vi "Z_MN_4952.vi"(4 "u":dbl format="%#_13g") -> (1 "y":dbl)   [LabVIEW 2019]
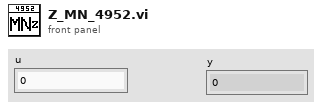
[diagram p1: front panel]
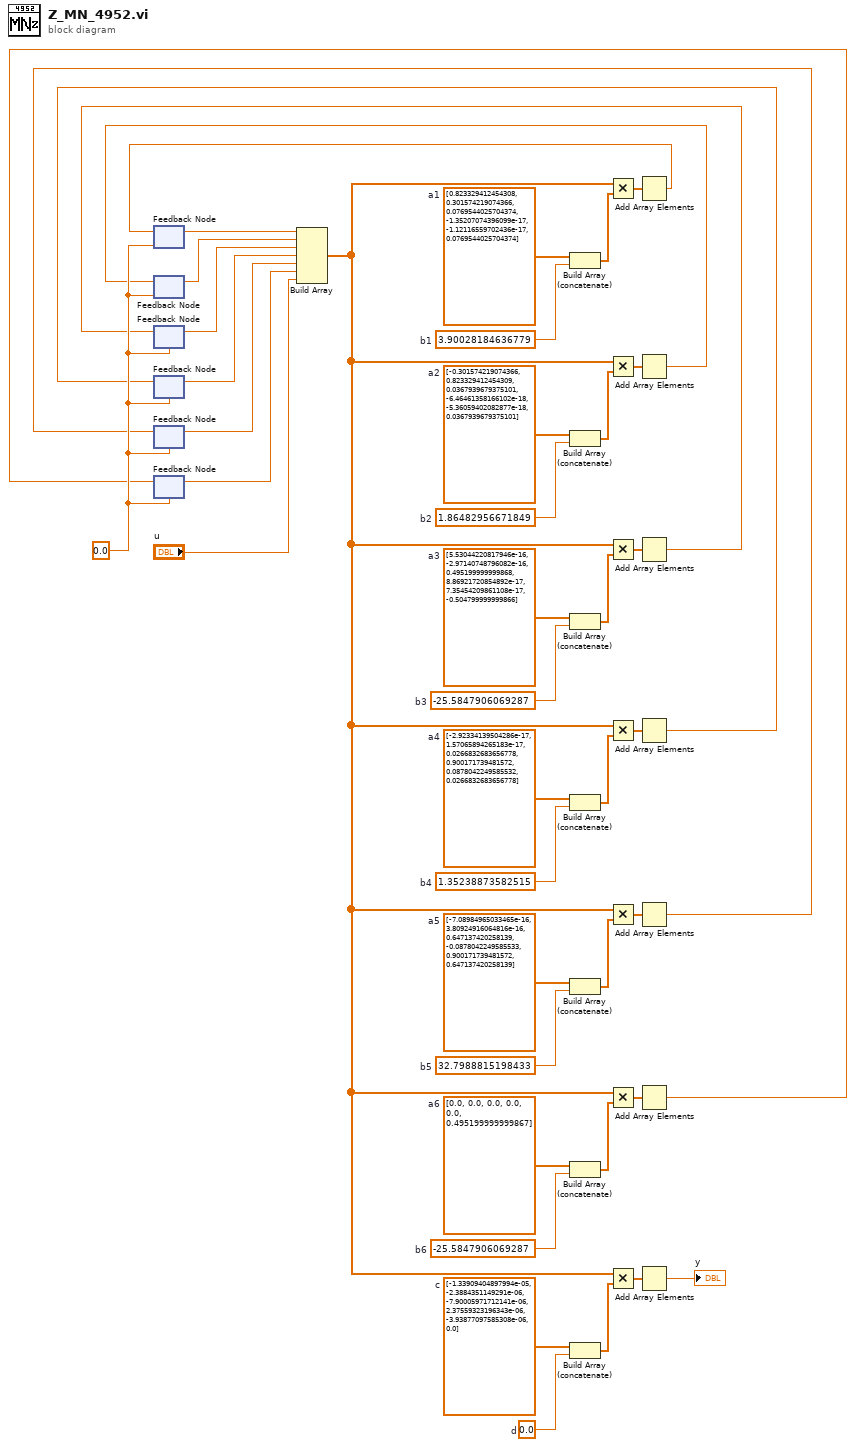
[diagram p0: block diagram]
diagram:
  w3 = 0.0  # d
  w2 = dbl[] [-1.33909404897994e-05, -2.3884351149291e-06, -7.90005971712141e-06, 2.37559323196343e-06, -3.93877097585308e-06, 0.0]  # c
  w5 = -25.5847906069287  # b6
  w6 = dbl[] [0.0, 0.0, 0.0, 0.0, 0.0, 0.495199999999867]  # a6
  w9 = 32.7988815198433  # b5
  w8 = dbl[] [-7.08984965033465e-16, 3.80924916064816e-16, 0.647137420258139, -0.0878042249585533, 0.900171739481572, 0.647137420258139]  # a5
  w11 = 1.35238873582515  # b4
  w12 = dbl[] [-2.92334139504286e-17, 1.57065894265183e-17, 0.0266832683656778, 0.900171739481572, 0.0878042249585532, 0.0266832683656778]  # a4
  w14 = -25.5847906069287  # b3
  w15 = dbl[] [5.53044220817946e-16, -2.97140748796082e-16, 0.495199999999868, 8.86921720854892e-17, 7.35454209861108e-17, -0.504799999999866]  # a3
  w18 = 1.86482956671849  # b2
  w17 = dbl[] [-0.301574219074366, 0.823329412454309, 0.0367939679375101, -6.46461358166102e-18, -5.36059402082877e-18, 0.0367939679375101]  # a2
  w20 = 3.90028184636779  # b1
  w21 = dbl[] [0.823329412454308, 0.301574219074366, 0.0769544025704374, -1.35207074396099e-17, -1.12116559702436e-17, 0.0769544025704374]  # a1
  w43 = 0.0
  n1 = feedback #1(w43) -> (w44:dbl)
  n2 = feedback #2(w43) -> (w42:dbl)
  n3 = feedback #3(w43) -> (w41:dbl)
  n4 = feedback #4(w43) -> (w40:dbl)
  n5 = feedback #5(w43) -> (w39:dbl)
  n6 = feedback #6(w43) -> (w38:dbl)
  n7 = Build Array(w44, w42, w41, w40, w39, w38, "u") -> (w33:dbl[])
  n8 = Build Array (concatenate)(w21, w20) -> (w19:dbl[])
  n9 = Build Array (concatenate)(w17, w18) -> (w16:dbl[])
  n10 = Build Array (concatenate)(w15, w14) -> (w13:dbl[])
  n11 = Build Array (concatenate)(w12, w11) -> (w10:dbl[])
  n12 = Build Array (concatenate)(w8, w9) -> (w7:dbl[])
  n13 = Build Array (concatenate)(w6, w5) -> (w4:dbl[])
  n14 = Build Array (concatenate)(w2, w3) -> (w1:dbl[])
  n15 = Multiply(x=w33, y=w19) -> (x*y=w35:dbl[])
  n16 = Multiply(x=w33, y=w16) -> (x*y=w32:dbl[])
  n17 = Multiply(x=w33, y=w13) -> (x*y=w31:dbl[])
  n18 = Multiply(x=w33, y=w10) -> (x*y=w30:dbl[])
  n19 = Multiply(x=w33, y=w7) -> (x*y=w29:dbl[])
  n20 = Multiply(x=w33, y=w4) -> (x*y=w28:dbl[])
  n21 = Multiply(x=w33, y=w1) -> (x*y=w37:dbl[])
  n22 = Add Array Elements(numeric array=w35) -> (sum=w27:dbl)
  n23 = feedback-in #1(w27) -> ()
  n24 = Add Array Elements(numeric array=w32) -> (sum=w26:dbl)
  n25 = feedback-in #2(w26) -> ()
  n26 = Add Array Elements(numeric array=w31) -> (sum=w25:dbl)
  n27 = feedback-in #3(w25) -> ()
  n28 = Add Array Elements(numeric array=w30) -> (sum=w24:dbl)
  n29 = feedback-in #4(w24) -> ()
  n30 = Add Array Elements(numeric array=w29) -> (sum=w23:dbl)
  n31 = feedback-in #5(w23) -> ()
  n32 = Add Array Elements(numeric array=w28) -> (sum=w22:dbl)
  n33 = feedback-in #6(w22) -> ()
  n34 = Add Array Elements(numeric array=w37) -> (sum=→"y":dbl)
